vi "MSG.vi"(8 "error in (no error)":errorcluster, 10 "Message":string) -> (0 "error out":errorcluster)   [LabVIEW 2018, in "MQTT Messages.lvlib"]
uses:
  MQTT Messages.lvlib
  MQTT_Singleton/MQTT_Singleton.lvlib
panel:
  out "JSON string":string
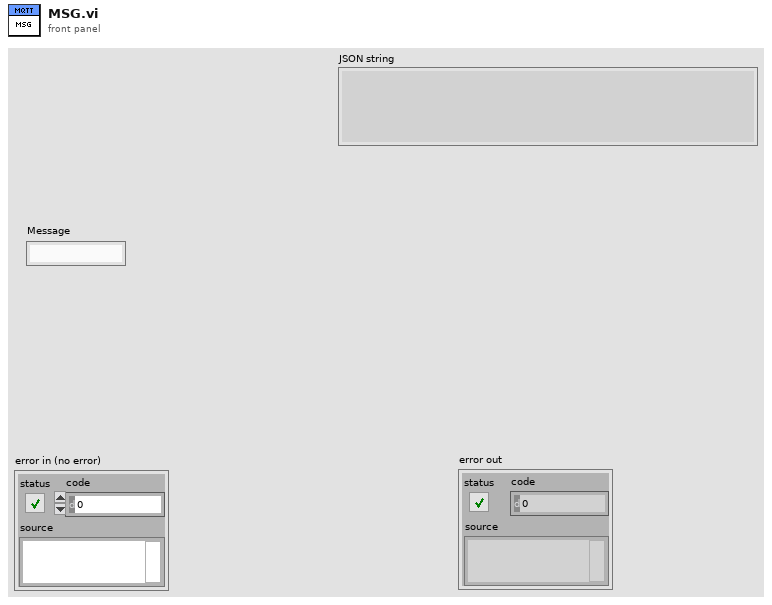
[diagram p1: front panel]
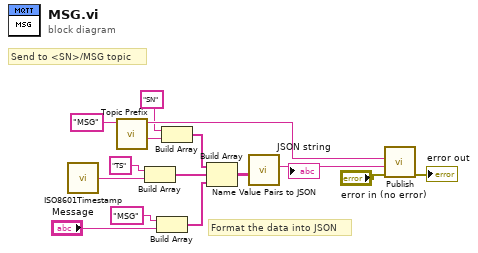
[diagram p0: block diagram]
diagram:
  # "Format the data into JSON"
  # "Send to <SN>/MSG topic"
  n1 = call "ISO8601Timestamp.vi"() -> ("date/time string"=w8:string)  [unwired: 5 in]
  n2 = call "Topic Prefix.vi"("Topic"="MSG" ("string")) -> ("SN"=w10:string, "Topic"=w12:string)  [unwired: 9 in]
  n3 = Build Array("TS" ("element"), w8) -> (w3:string[])
  n4 = Build Array("MSG" ("element"), "Message") -> (w2:string[])
  n5 = Build Array("SN" ("element"), w10) -> (w4:string[])
  n6 = Build Array(w4, w3, w2) -> (w1:string[][])
  n7 = call "Name Value Pairs to JSON.vi"("Message"=w1) -> ("JSON string"=w11:string)  [unwired: 10 in]
  "JSON string" <- w11
  n8 = call "Publish.vi"("error in (no error)"="error in (no error)", "Message"=w11, "Topic"=w12) -> ("error out"=→"error out":errorcluster)  [unwired: 8 in]
